vi "Asynchronous - Update Acyclic Labels Parameters Channels.vi"(5 "Channel Data []":T5[](array[typedef])=[{"Labels Settings"=[{"Name"="", "xmlName"="", "Label"=0, "transferPeriod"=0, "SDI_Enabled"=FALSE, "SDI"=0, "Word"={"Param Setting"={"Start Bit"=[], "Num Bits"=[], "Signed?"=[], "ScaleFac"=[], "ScaleOffset"=[], "Block Data Refs"=[], "Encoding"=[], "Values Array"=[], "Item Refs"=[]}}, "TransferType"=enum."ScheduledLabel", "has timestamp?"=FALSE, "Label Disable/Trigger Channel Reference"=0, "Message Handle"=0, "Initialized?"=FALSE, "Word Initial Raw Value"=0, "Label Timestamp Channel Data Reference"=0}], "channel handle"=0, "channel #"=0}] {"Labels Settings"."Label Timestamp Channel Data Reference" format="%.0x"; "Labels Settings"."Label Disable/Trigger Channel Reference" format="%.0x"; "Labels Settings"."Word"."Param Setting"."Item Refs" format="%.0x"; "Labels Settings"."Word"."Param Setting"."Num Bits" min=1 max=32; "Labels Settings"."Word"."Param Setting"."Start Bit" min=8 max=31; "Labels Settings"."Label" format="%.0o"}, 7 "Map":T4[](array[typedef]) {"Channel Data Reference" format="%.0x"}, 8 "Error (in)":errorcluster, 9 "Updated FIFO Index []":i32[](array[numeric]), 10 "Doubles []":dbl[](array[numeric]), 11 "Raw Values":T1) -> (0 "Error (out)":errorcluster, 4 "Raw Values Array":u32[](array[numeric]), 6 "Raw Value Index":i32[](array[numeric]))   [LabVIEW 2020, in "Ballard Arinc-429 Engine.lvlib"]
uses:
  Ballard Arinc-429 Engine.lvlib
  Shared/Controls and Global/RT HW Channel.ctl
  Shared/Controls and Global/RT Label Settings.ctl
  Shared/Controls and Global/Label.ctl
  Shared/Controls and Global/transferPeriod.ctl
  Shared/Controls and Global/RT Word Settings.ctl
  Shared/Controls and Global/RT Param Setting.ctl
  Shared/Controls and Global/Start Bit.ctl
  Shared/Controls and Global/Number of Bits.ctl
  <vilib>/NI VeriStand/Custom Device API/Block Data Reference.ctl
  <vilib>/NI VeriStand/Custom Device API/Data Reference.ctl
  <vilib>/NI VeriStand/Custom Device API/Custom Device Item Ref.ctl
  Shared/Controls and Global/TransferType.ctl
  RT Controls/RT Tx Association.ctl
  RT Controls/RT Tx Default Raw Value.ctl
  RT Controls/RT Tx Default Raw Value_Association.ctl
  Insert BCD Parameter.vi
  <instrlib>/BTI429Lib/BTI429LV.lvlib
  <vilib>/NI VeriStand/Custom Device Tools/Custom Device Utility Library/Custom Device Utility Library.lvlib
  Shared/Ballard Arinc-429 Shared.lvlib
  <vilib>/NI VeriStand/Custom Device API/Custom Device API.lvlib
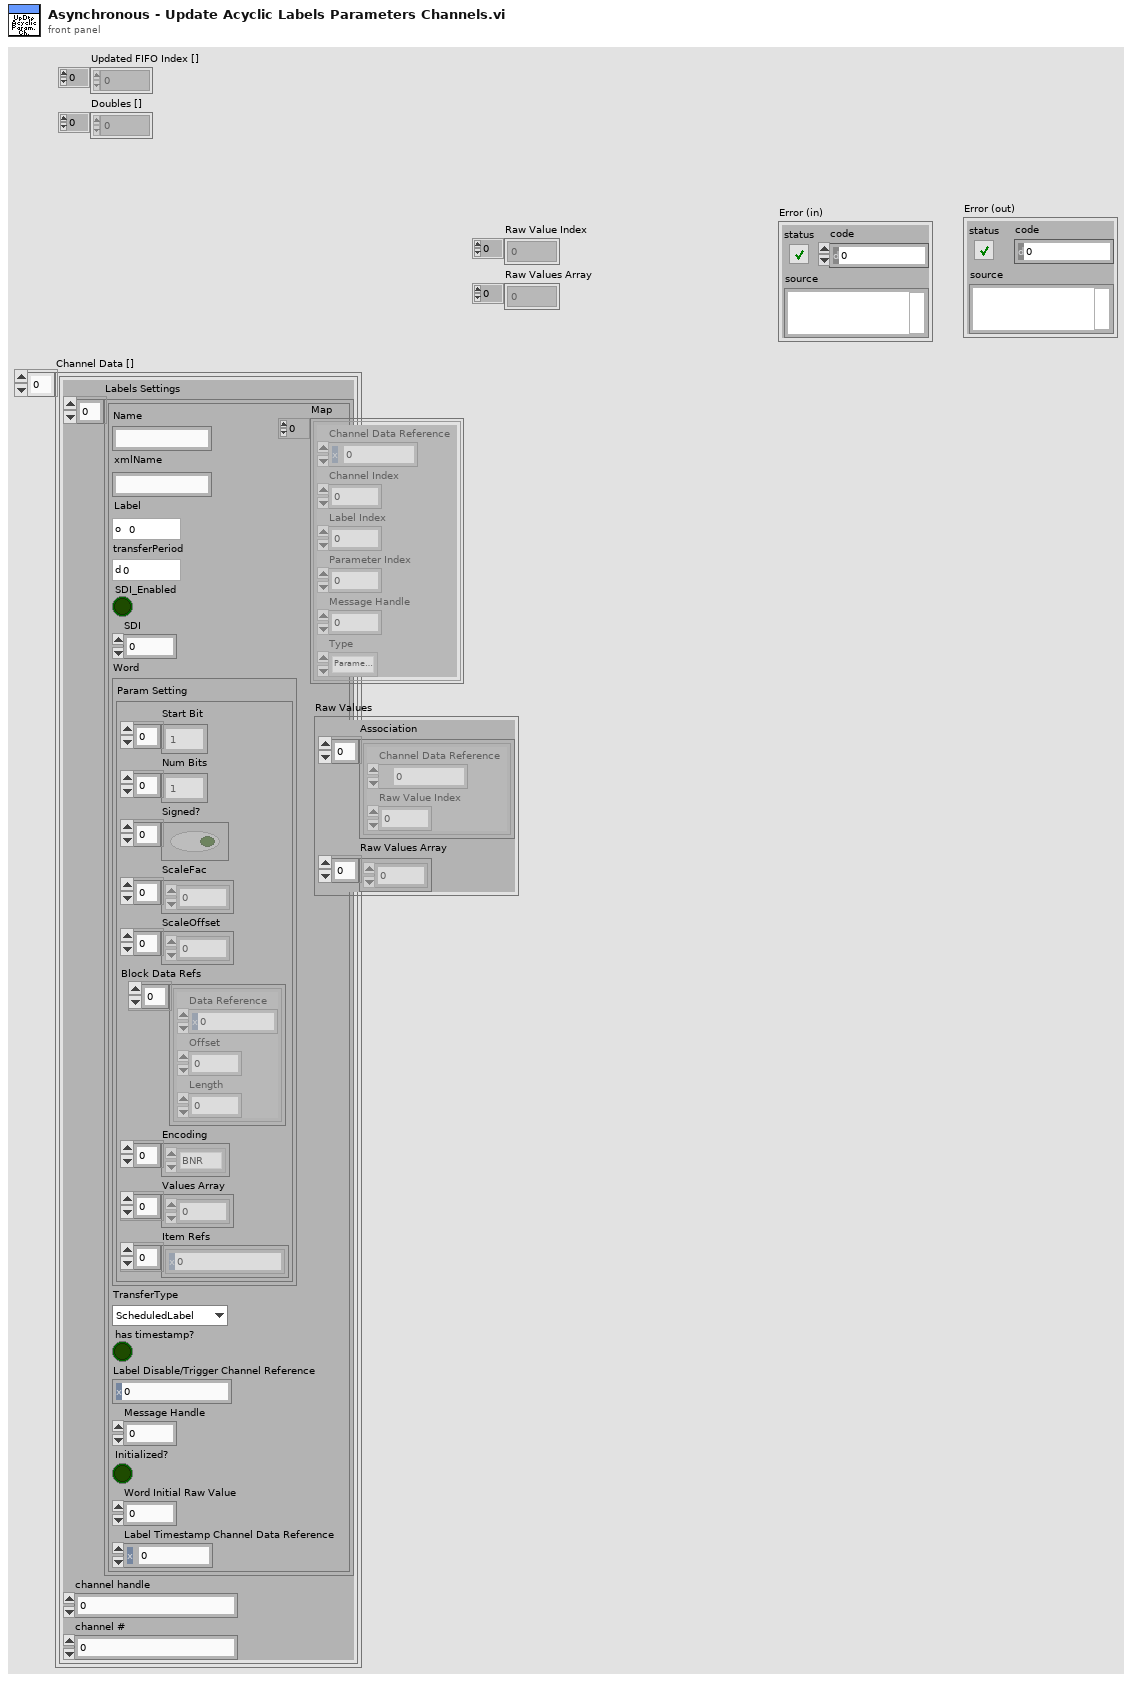
[diagram p1: front panel]
types:
  T1 = typedef "Ballard Arinc-429 Engine.lvlib/RT Tx Default Raw Value.ctl" = cluster{"Association":T2[], "Raw Values Array":u32[]}
  T2 = typedef "Ballard Arinc-429 Engine.lvlib/RT Tx Default Raw Value_Association.ctl" = cluster{"Channel Data Reference":T3, "Raw Value Index":i32}
  T3 = typedef "Custom Device API.lvlib/Data Reference.ctl" = i32
  T4 = typedef "Ballard Arinc-429 Engine.lvlib/RT Tx Association.ctl" = cluster{"Channel Data Reference":T3, "Channel Index":i32, "Label Index":i32, "Parameter Index":i32, "Message Handle":u64, "Type":enum16{"Parameter Channel", "Disable/Trigger Channel"}}
  T5 = typedef "Ballard Arinc-429 Shared.lvlib/RT HW Channel.ctl" = cluster{"Labels Settings":T6[], "channel handle":u64, "channel #":u16}
  T6 = typedef "Ballard Arinc-429 Shared.lvlib/RT Label Settings.ctl" = cluster{"Name":string, "xmlName":string, "Label":T7, "transferPeriod":T8, "SDI_Enabled":bool, "SDI":u8, "Word":T9, "TransferType":T15, "has timestamp?":bool, "Label Disable/Trigger Channel Reference":T14, "Message Handle":u64, "Initialized?":bool, "Word Initial Raw Value":u32, "Label Timestamp Channel Data Reference":T3}
  T7 = typedef "Ballard Arinc-429 Shared.lvlib/Label.ctl" = u8
  T8 = typedef "Ballard Arinc-429 Shared.lvlib/transferPeriod.ctl" = u32
  T9 = typedef "Ballard Arinc-429 Shared.lvlib/RT Word Settings.ctl" = cluster{"Param Setting":T10}
  T10 = typedef "Ballard Arinc-429 Shared.lvlib/RT Param Setting.ctl" = cluster{"Start Bit":T11[], "Num Bits":T12[], "Signed?":bool[], "ScaleFac":dbl[], "ScaleOffset":dbl[], "Block Data Refs":T13[], "Encoding":enum16{"BNR", "BCD", "Discrete"}[], "Values Array":dbl[], "Item Refs":T14[]}
  T11 = typedef "Ballard Arinc-429 Shared.lvlib/Start Bit.ctl" = i32
  T12 = typedef "Ballard Arinc-429 Shared.lvlib/Number of Bits.ctl" = i32
  T13 = typedef "Custom Device API.lvlib/Block Data Reference.ctl" = cluster{"Data Reference":T3, "Offset":u64, "Length":u64}
  T14 = typedef "Custom Device API.lvlib/Custom Device Item Ref.ctl" = u64
  T15 = typedef "Ballard Arinc-429 Shared.lvlib/TransferType.ctl" = enum16{"ScheduledLabel", "Acyclic", "Block", "Strobe"}
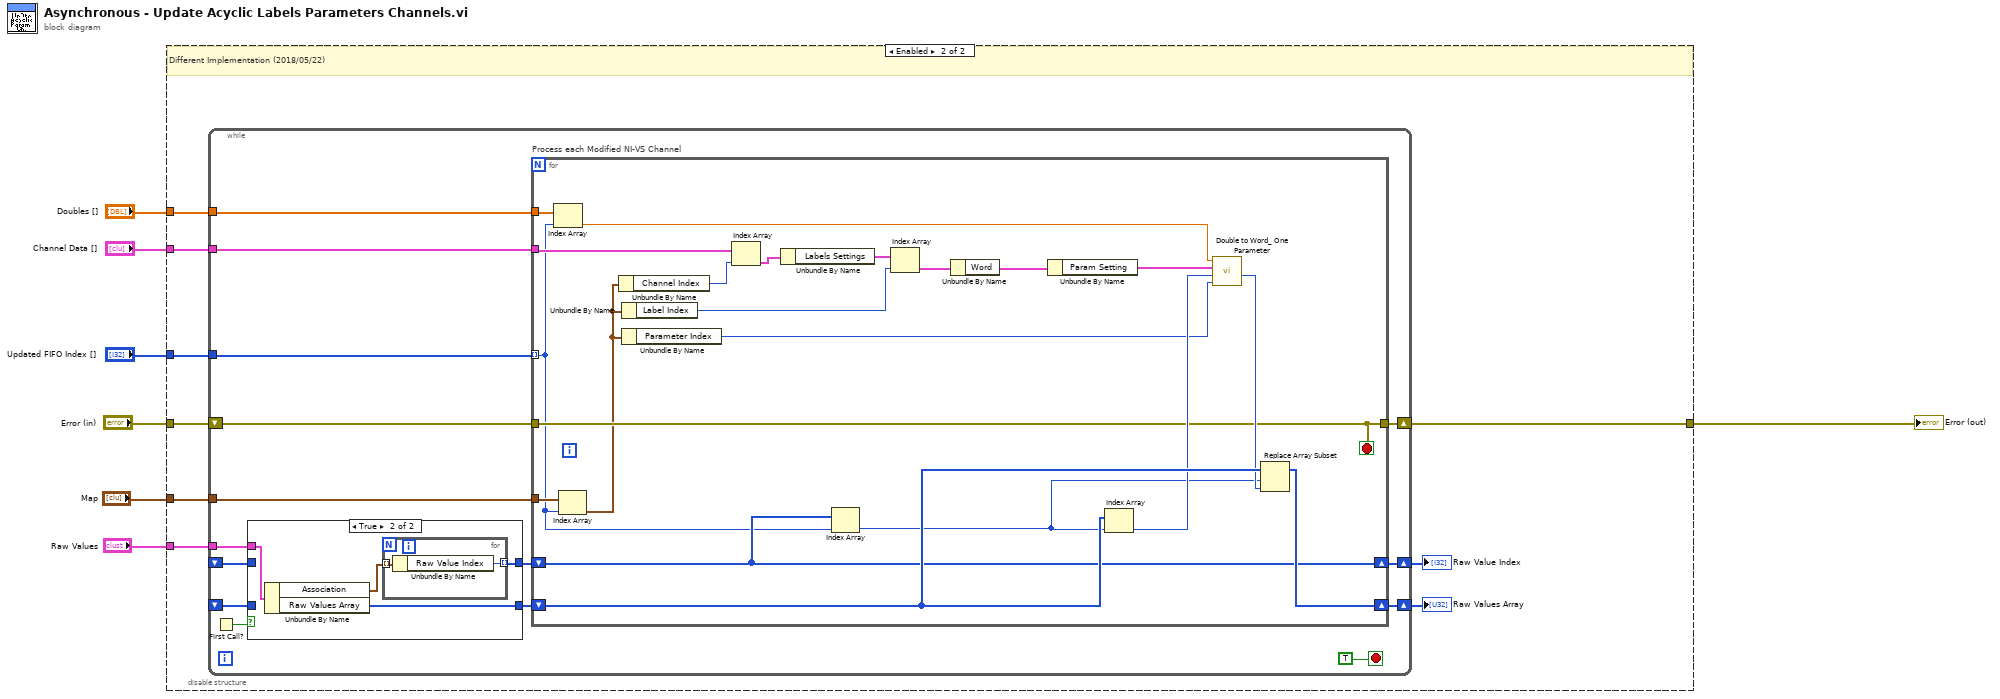
[diagram p0: block diagram]
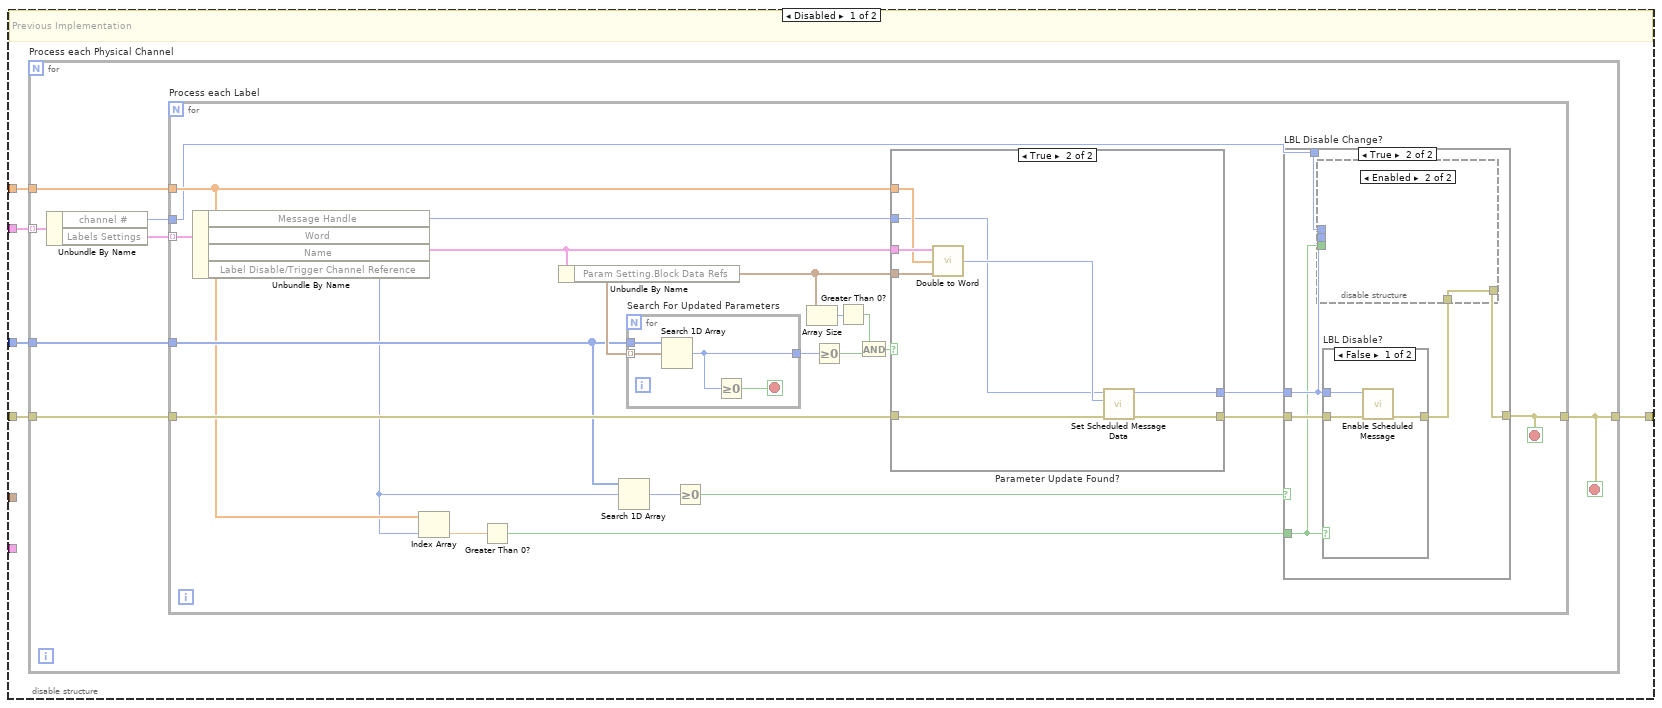
[diagram p2: hidden frame]
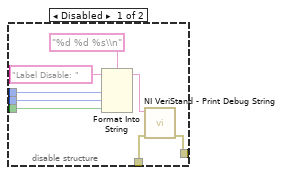
[diagram p4: hidden frame]
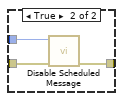
[diagram p5: hidden frame]
diagram:
  n1 = disable-structure shown="Enabled" {
    disable-tunnel: "Channel Data []" -> [w12 w85]
    disable-tunnel: "Updated FIFO Index []" -> [w11 w84]
    disable-tunnel: "Error (in)" -> [w10 w83]
    disable-tunnel: [w9 w82] -> w4
    disable-tunnel: "Doubles []" -> [w8 w81]
    disable-tunnel: "Map" -> [_ w80]
    disable-tunnel: "Raw Values" -> [_ w79]
    frame Disabled {
      # "Previous Implementation"
      n2 = for "Process each Physical Channel" {
        tunnel: w12 -> [w19] mode=indexing
        tunnel: w11 -> [w17]
        tunnel: w8 -> [w16]
        tunnel: w10 -> [w15]
        tunnel: [w14] -> w9
        stop <- w14 stop-if-true
        n3 = Unbundle By Name(w19) -> ("channel #"=w13:u16, "Labels Settings"=w18:T6[])
        n4 = for "Process each Label" {
          tunnel: w18 -> [w40] mode=indexing
          tunnel: w17 -> [w32]
          tunnel: w16 -> [w27]
          tunnel: [w29] -> w14
          tunnel: w15 -> [w38]
          tunnel: w13 -> [w21]
          stop <- w29 stop-if-true
          n5 = Unbundle By Name(w40) -> ("Message Handle"=w22:u64, "Word"=w20:T9, "Label Disable/Trigger Channel Reference"=w26:T14)  [unwired: 1 out]
          n6 = Index Array(array=w27, index=w26) -> (element=w25:dbl)
          n7 = Greater Than 0?(x=w25) -> (x > 0?=w24:bool)
          n8 = Unbundle By Name(w20) -> ("Param Setting.Block Data Refs"=w37:T13[])
          n9 = Search 1D Array(1D array=w32, element=w26) -> (index of element=w31:i32)  [unwired: 1 in]
          n10 = for "Search For Updated Parameters" {
            tunnel: w32 -> [w76]
            tunnel: w37 -> [w75] mode=indexing
            tunnel: [w74] -> w39
            stop <- w73 stop-if-true
            n11 = Search 1D Array(1D array=w76, element=w75) -> (index of element=w74:i32)  [unwired: 1 in]
            n12 = Greater Or Equal To 0?(x=w74) -> (x >= 0?=w73:bool)
          }
          n13 = Greater Or Equal To 0?(x=w31) -> (x >= 0?=w30:bool)
          n14 = Array Size(array=w37) -> (size(s)=w36:i32)
          n15 = Greater Or Equal To 0?(x=w39) -> (x >= 0?=w34:bool)
          n16 = Greater Than 0?(x=w36) -> (x > 0?=w35:bool)
          n17 = And(x=w35, y=w34) -> (x .and. y?=w33:bool)
          n18 = case "Parameter Update Found?" shown="True" w33 {
            tunnel: w27 -> [_ w68]
            tunnel: w20 -> [_ w72]
            tunnel: w38 -> [w64 w67]
            tunnel: [w64 w71] -> w28
            tunnel: w37 -> [_ w69]
            tunnel: w22 -> [w63 w66]
            tunnel: [w63 w65] -> w23
            frame False {
            }
            frame True {
              n19 = call "Double to Word.vi"("Word"=w72, "Doubles In []"=w68, "Channel FIFO Buffer Index"=w69) -> ("Word"=w70:u32)  [unwired: 12 in]
              n20 = call <instrlib>:"Set Scheduled Message Data.vi"("error in (no error)"=w67, "value"=w70, "message handle in"=w66) -> ("error out"=w71:errorcluster, "message handle out"=w65:u64)  [unwired: 7 in]
            }
          }
          n21 = case "LBL Disable Change?" shown="True" w30 {
            tunnel: [w41 w46] -> w29
            tunnel: w28 -> [w41 w47]
            tunnel: w24 -> [_ w42]
            tunnel: w23 -> [_ w43]
            tunnel: w21 -> [_ w44]
            frame False {
            }
            frame True {
              n22 = case "LBL Disable?" shown="False" w42 {
                tunnel: [w59 w62] -> w45
                tunnel: w47 -> [w58 w61]
                tunnel: w43 -> [w57 w60]
                frame False {
                  n23 = call <instrlib>:"Enable Scheduled Message.vi"("error in (no error)"=w58, "message handle in"=w57) -> ("error out"=w59:errorcluster)  [unwired: 8 in, 1 out]
                }
                frame True {
                  n24 = call <instrlib>:"Disable Scheduled Message.vi"("error in (no error)"=w61, "message handle in"=w60) -> ("error out"=w62:errorcluster)  [unwired: 8 in, 1 out]
                }
              }
              n25 = disable-structure shown="Enabled" {
                disable-tunnel: [w55 w56] -> w46
                disable-tunnel: w45 -> [w54 w56]
                disable-tunnel: w44 -> [w51 _]
                disable-tunnel: w43 -> [w50 _]
                disable-tunnel: w42 -> [w49 _]
                frame Disabled {
                  n26 = Format Into String(format string="%d %d %s\\n", initial string="Label Disable: ", w51, w50, w49) -> (resulting string=w52:string)  [unwired: 1 in, 1 out]
                  n27 = call <vilib>:"NI VeriStand - Print Debug String.vi"("error in (no error)"=w54, "Message"=w52) -> ("error out"=w55:errorcluster)  [unwired: 9 in]
                }
                frame Enabled {
                }
              }
            }
          }
        }
      }
    }
    frame Enabled {
      # "Different Implementation (2018/05/22)"
      n28 = while {
        tunnel: w85 -> [w100]
        tunnel: w84 -> [w99]
        tunnel: w81 -> [w96]
        tunnel: w80 -> [w95]
        shift-right: [w97] -> w82
        shift-left: w83 -> [w98]
        tunnel: w79 -> [w93]
        shift-right: [w91] -> w77
        shift-left: _ -> [w90]
        shift-right: [w88] -> w78
        shift-left: _ -> [w87]
        stop <- TRUE stop-if-true
        n29 = First Call?() -> (First Call?: T/F=w86:bool)
        n30 = case shown="True" w86 {
          tunnel: w93 -> [_ w106]
          tunnel: [w102 w105] -> w92
          tunnel: w90 -> [w102 _]
          tunnel: [w101 w103] -> w89
          tunnel: w87 -> [w101 _]
          frame False {
          }
          frame True {
            n31 = Unbundle By Name(w106) -> ("Association"=w104:T2[], "Raw Values Array"=w105:u32[])
            n32 = for {
              tunnel: w104 -> [w108] mode=indexing
              tunnel: [w107] -> w103 mode=indexing
              n33 = Unbundle By Name(w108) -> ("Raw Value Index"=w107:i32)
            }
          }
        }
        n34 = for "Process each Modified NI-VS Channel" {
          tunnel: w100 -> [w129]
          tunnel: w99 -> [w110] mode=indexing
          tunnel: w96 -> [w123]
          tunnel: w98 -> [w116]
          tunnel: [w116] -> w97
          tunnel: w95 -> [w125]
          shift-right: [w120] -> w91
          shift-left: w92 -> [w121]
          shift-right: [w111] -> w88
          shift-left: w89 -> [w111]
          stop <- w116 stop-if-true
          n35 = Index Array(array=w123, index=w110) -> (element=w122:dbl)
          n36 = Index Array(array=w125, index=w110) -> (element=w113:T4)
          n37 = Unbundle By Name(w113) -> ("Channel Index"=w115:i32)
          n38 = Unbundle By Name(w113) -> ("Label Index"=w114:i32)
          n39 = Unbundle By Name(w113) -> ("Parameter Index"=w112:i32)
          n40 = Index Array(array=w129, index=w115) -> (element=w128:T5)
          n41 = Unbundle By Name(w128) -> ("Labels Settings"=w127:T6[])
          n42 = Index Array(array=w111, index=w110) -> (element=w109:i32)
          n43 = Index Array(array=w127, index=w114) -> (element=w126:T6)
          n44 = Unbundle By Name(w126) -> ("Word"=w124:T9)
          n45 = Unbundle By Name(w124) -> ("Param Setting"=w118:T10)
          n46 = Index Array(array=w121, index=w109) -> (element=w117:u32)
          n47 = call "Double to Word_ One Parameter.vi"("Parameter Index"=w112, "Word In"=w117, "Param Setting"=w118, "NI-VS Channel"=w122) -> ("Word Out"=w119:u32)  [unwired: 5 in]
          n48 = Replace Array Subset(array=w121, new element=w119, index=w109) -> (w120:u32[])
        }
      }
      "Raw Value Index" <- w78
      "Raw Values Array" <- w77
    }
  }
  "Error (out)" <- w4
